vi "SelectChanCurveRef.vi"(8 "错误输入（无错误）":errorcluster) -> (0 "错误输出":errorcluster, 3 "返回值":i32)   [LabVIEW 2014]
uses:
  ZXUTConfigMgr.dll
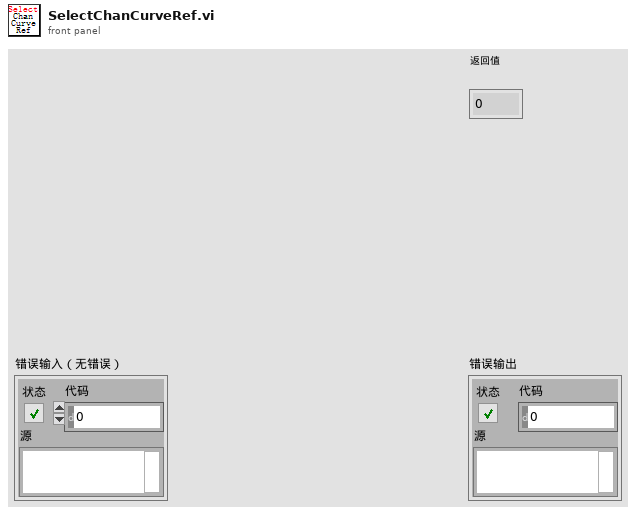
[diagram p1: front panel]
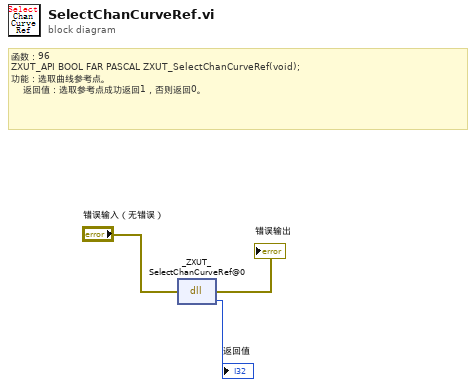
[diagram p0: block diagram]
diagram:
  # "函数：96\nZXUT_API BOOL\tFAR PASCAL ZXUT_SelectChanCurveRef(void);\n功能：选取曲线参考点。\n\t   返回值：选取参考点成功返回1，否则返回0。"
  n1 = dll-call lib="PTH2eabs D软件超声实时监测软件ZXUTAppDemo(华南理工V02.00)X86DllZXUTConfigMgr.dll" fn="_ZXUT_SelectChanCurveRef@0"(error in="错误输入（无错误）") -> (error out=→"错误输出":errorcluster, "返回值"=→"返回值":i32)  [unwired: 2 in, 1 out]
